vi "joystick_to_angle.vi"(8 "y":dbl, 9 "x":dbl) -> (1 "Theta":dbl)   [LabVIEW 2020]
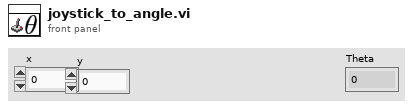
[diagram p1: front panel]
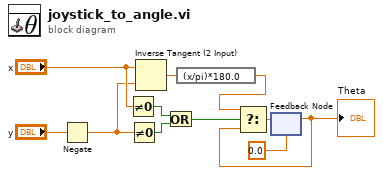
[diagram p0: block diagram]
diagram:
  n1 = Negate(x="y") -> (-x=w1:dbl)
  n2 = Not Equal To 0?(x="x") -> (x != 0?=w6:bool)
  n3 = Not Equal To 0?(x=w1) -> (x != 0?=w5:bool)
  n4 = Inverse Tangent (2 Input)(1:w1, 2:"x") -> (0:w4:dbl)
  n5 = Or(x=w6, y=w5) -> (x .or. y?=w9:bool)
  n6 = expression code="(x/pi)*180.0" ("radians to degrees")(w4) -> (w10:dbl)
  n7 = feedback #1(0.0 ("angle out")) -> (w11:dbl)
  "Theta" <- w11
  n8 = Select(t=w10, s=w9, f=w11) -> (s? t:f=w7:dbl)
  n9 = feedback-in #1(w7) -> ()
